vi "Measure.vi"(0 "Yokogawa WT2X0 in":refnum<class "Yokogawa WT2X0.lvclass">, 1 "Card Number":u8=1 min=1 step=1, 5 "Measurement Type":T1, 7 "Preset (2: Preset 2)":u16(ring)=2 items=["", "Preset1", "Preset2", "Preset3", "Preset4"], 9 "Number of Item (255)":i32=255 min=1 max=255 step=1, 11 "error in (no error)":errorcluster) -> (4 "Yokogawa WT2X0 out":refnum<class "Yokogawa WT2X0.lvclass">, 8 "Array":dbl[](array[numeric]), 15 "error out":errorcluster)   [LabVIEW 2012, in "Universal Power Meter.lvlib" / "Yokogawa WT2X0.lvlib" / "Yokogawa WT2X0.lvclass"]
uses:
  Yokogawa WT2X0.lvclass
  Universal Power Meter class/Master Control.ctl
  Universal Power Meter class/Universal Power Meter.lvclass
panel:
  out "Full Array":string[][](array[string])
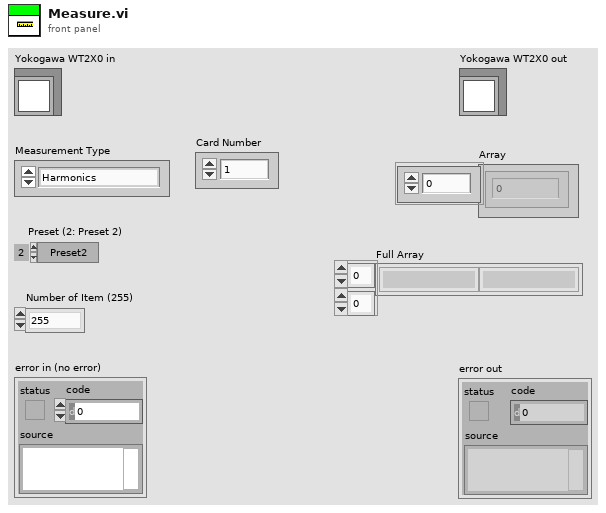
[diagram p1: front panel]
types:
  T1 = typedef "Universal Power Meter.lvlib/Universal Power Meter.lvclass/Master Control.ctl" = enum16{"Harmonics", "RMS"}
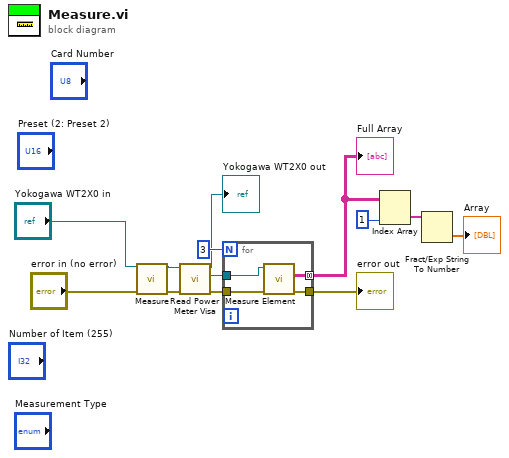
[diagram p0: block diagram]
diagram:
  n1 = call-parent "Measure.vi"("Universal Power Meter in"="Yokogawa WT2X0 in", "error in (no error)"="error in (no error)") -> ("Universal Power Meter out"=w11:refnum<class "Yokogawa WT2X0.lvclass">, "error out"=w10:errorcluster)  [unwired: 11 in, 1 out]
  n2 = call "Read Power Meter Visa.vi"("error in (no error)"=w10, "Universal Power Meter in"=w11) -> ("error out"=w5:errorcluster, "Power Meter Visa"=w9:refnum<visa-resource-name>, "Universal Power Meter out"=→"Yokogawa WT2X0 out":refnum<class "Yokogawa WT2X0.lvclass">)  [unwired: 7 in]
  n3 = for {
    N: 3 -> [_]
    tunnel: w9 -> [w17]
    tunnel: [w16] -> w6 mode=concatenating
    tunnel: w5 -> [w15]
    tunnel: [w14] -> w4
    n4 = call "Measure Element.vi"("error in (no error)"=w15, "VISA resource name"=w17) -> ("error out"=w14:errorcluster, "Array"=w16:string[][])  [unwired: 7 in, 1 out]
  }
  "error out" <- w4
  "Full Array" <- w6
  n5 = Index Array(array=w6, index (col)=1 ("disabled index (col)")) -> (element=w2:string[])  [unwired: 1 in]
  n6 = Fract/Exp String To Number(string=w2) -> (number=→"Array":dbl[])  [unwired: 3 in, 1 out]
